vi "Get number of Calls.vi"(8 "error in (no error)":errorcluster, 11 "Mock Filter in":refnum<class "Mock Filter.lvclass">) -> (0 "error out":errorcluster, 2 "Number of Calls":i32, 3 "Mock Filter out":refnum<class "Mock Filter.lvclass">)   [LabVIEW 2020, in "Mock Filter.lvclass"]
uses:
  Mock Filter.lvclass
  Mock Filter.lvclass/Mock Filter.ctl
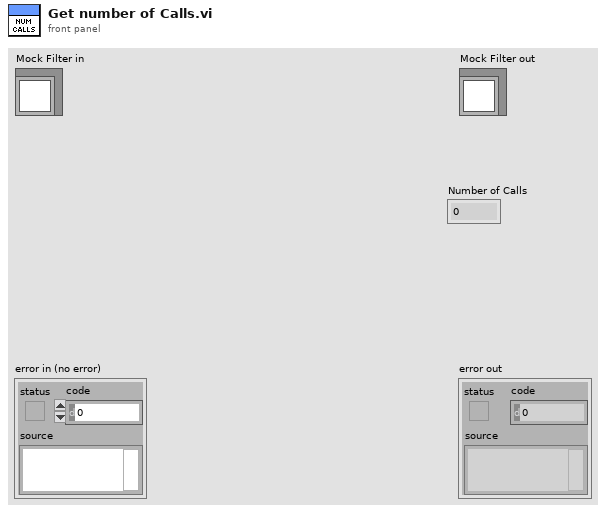
[diagram p1: front panel]
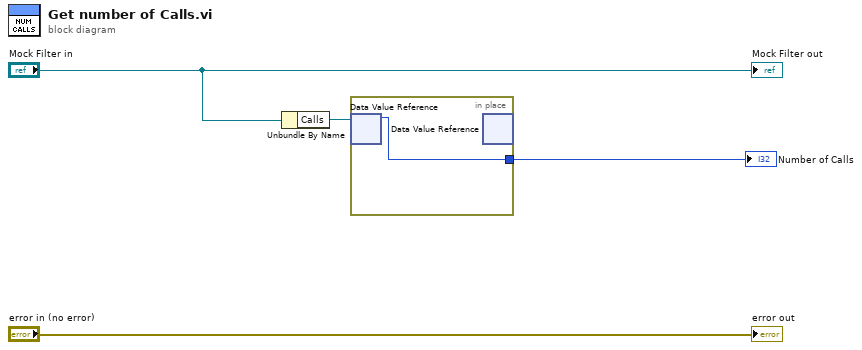
[diagram p0: block diagram]
diagram:
  n1 = Unbundle By Name("Mock Filter in") -> ("Calls"=w2:refnum<data-value>)
  n2 = in-place {
    in-place-border: [w5] -> w1
    n3 = in-place-dvr #1(w2) -> (w5:i32)  [unwired: 1 out]
    n4 = in-place-dvr #1() -> ()  [unwired: 1 in, 2 out]
  }
  "Number of Calls" <- w1
  "error out" <- "error in (no error)"
  "Mock Filter out" <- "Mock Filter in"
